vi "Shutdown.vi"(8 "error in (no error)":errorcluster, 10 "Reply Channel":refnum<notifier>, 11 "Actor in":refnum<class "Actor.lvclass">) -> (0 "error out":errorcluster, 3 "Actor out":refnum<class "Actor.lvclass">)   [LabVIEW 2015, in "Actor.lvclass"]
uses:
  Actor.lvclass
  Messaging/Message/Message.lvclass
  Actor.lvclass/Actor.ctl
  Messaging/Message/Message.lvclass/Message.ctl
  Utility/Utility.lvlib
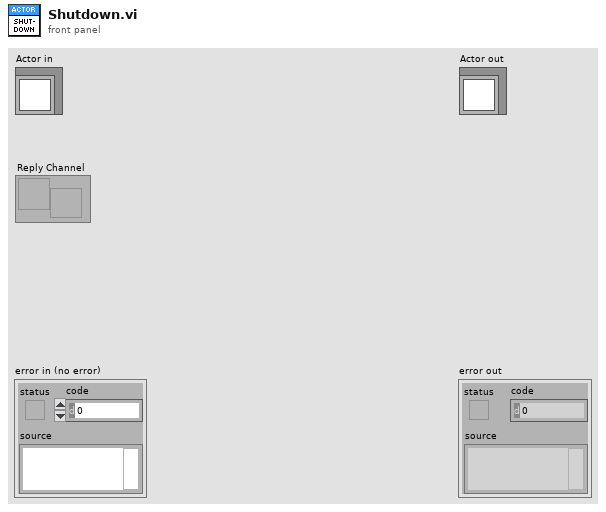
[diagram p1: front panel]
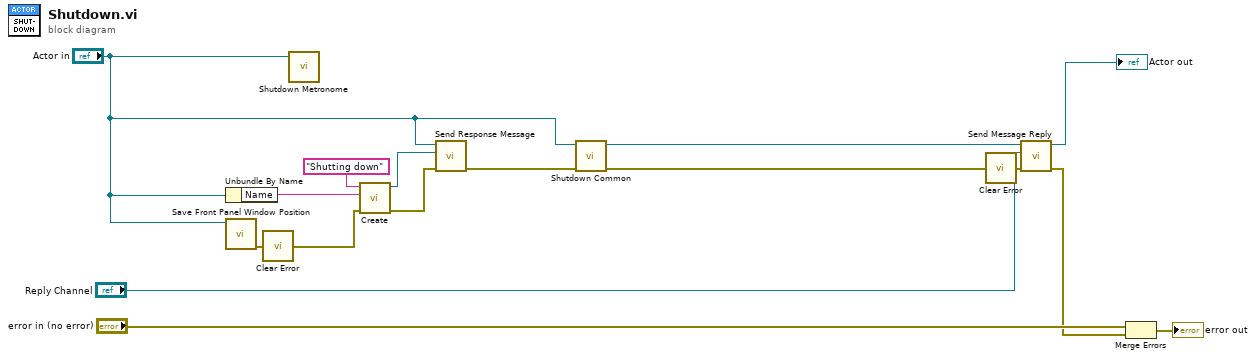
[diagram p0: block diagram]
diagram:
  n1 = Unbundle By Name("Actor in") -> ("Name"=w7:string)
  n2 = call "Save Front Panel Window Position.vi"("Actor in"="Actor in") -> ("error out"=w3:errorcluster)  [unwired: 10 in]
  n3 = call "Clear Error.vi"("error in (no error)"=w3) -> ("error out"=w2:errorcluster)
  n4 = call "Shutdown Metronome.vi"("Actor in"="Actor in") -> ()  [unwired: 11 in]
  n5 = call "Create.vi"("error in (no error)"=w2, "Data"=w7, "Name"="Shutting down" ("format string")) -> ("error out"=w12:errorcluster, "Message out"=w8:refnum<class "Message.lvclass">)  [unwired: 7 in]
  n6 = call-dynamic "Send Response Message.vi"("error in (no error)"=w12, "Message"=w8, "Actor in"="Actor in") -> ("error out"=w11:errorcluster)  [unwired: 8 in]
  n7 = call "Shutdown Common.vi"("error in (no error)"=w11, "Actor in"="Actor in") -> ("error out"=w16:errorcluster, "Actor out"=w10:refnum<class "Actor.lvclass">)  [unwired: 8 in]
  n8 = call "Clear Error.vi"("error in (no error)"=w16) -> ("error out"=w9:errorcluster)
  n9 = call-dynamic "Send Message Reply.vi"("error in (no error)"=w9, "Reply Channel"="Reply Channel", "Actor in"=w10) -> ("error out"=w5:errorcluster, "Actor out"=→"Actor out":refnum<class "Actor.lvclass">)  [unwired: 7 in]
  n10 = Merge Errors("error in (no error)", w5) -> (→"error out":errorcluster)
